vi "EF_GetFeaturesVectorScalogram.vi"(7 "TimeShiftsNum":dbl=50.0, 8 "ChannelNumber":i32=-1, 9 "High cutoff frequency":dbl, 10 "Low cutoff frequency":dbl, 11 "Array Of Waveforms in":waveform(dbl)[](array[waveform])) -> (0 "StackedSpectra":dbl[][](array[numeric]), 2 "size(s)":i32[](array[numeric]), 3 "StackedScalograms":dbl[][](array[numeric]))   [LabVIEW 2016, in "Feature Extraction.lvlib"]
uses:
  <vilib>/Analysis/baseanly.llb/Mean (DBL).vi
  <vilib>/addons/Wavelet Analysis/continuous wavelet transform.llb/WA Analytic Wavelet Transform (Waveform).vi
  Feature Extraction.lvlib
  <vilib>/addons/_Advanced Signal Processing/NI_AdvSigProcTFA.lvlib
  <vilib>/addons/_Advanced Signal Processing/NI_AdvSigProcWA.lvlib
  <vilib>/Analysis/NI_AALBase.lvlib
panel:
  out "Энергетический спектр сигнала ЭЭГ":dbl[](graph)
  out "Сигнал ЭЭГ":waveform(dbl)(graph)
  out "Матрица квадратов коэффициентов вейвлет-разложения":dbl[][](graph)
  # "This VI is a part of BCI Design library, http://www.ru-bci.org \nCopyright © 2020, Sotnikov Peter, All rights reserved. License: GNU GPLv3"
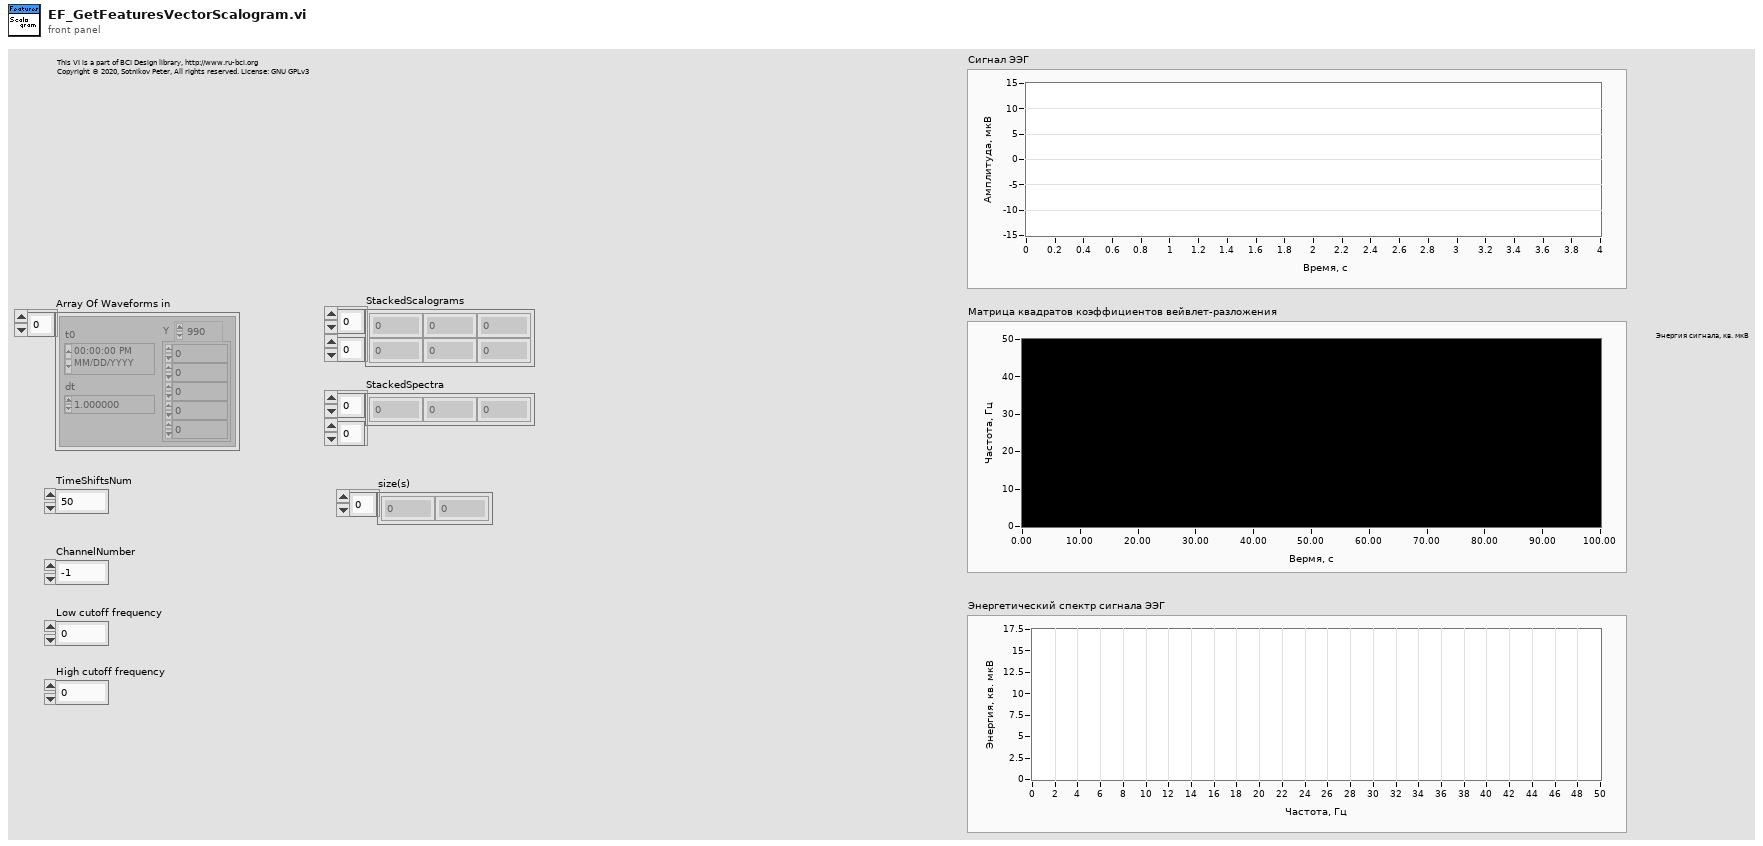
[diagram p1: front panel]
types:
  T1 = cluster{"frequency offset":dbl, "frequency multiplier":dbl}
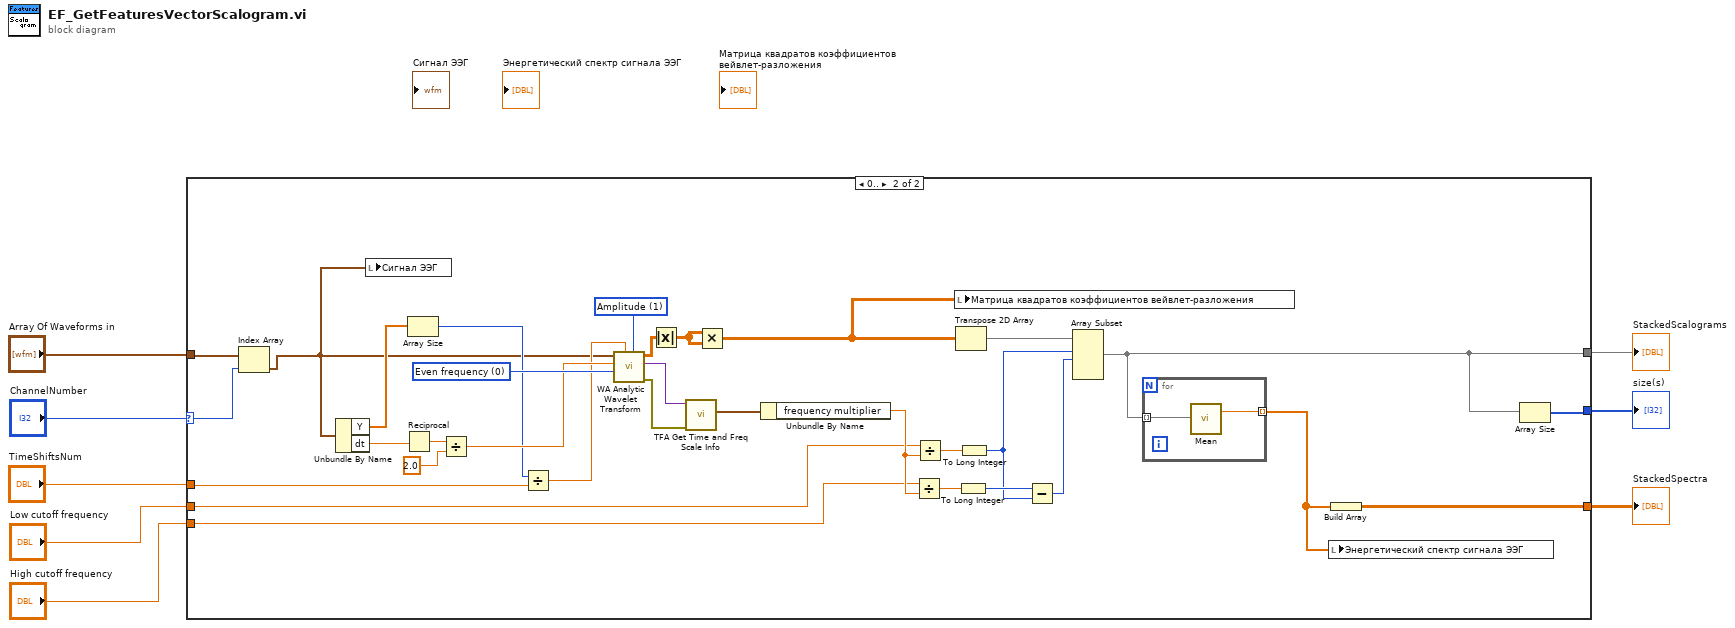
[diagram p0: block diagram]
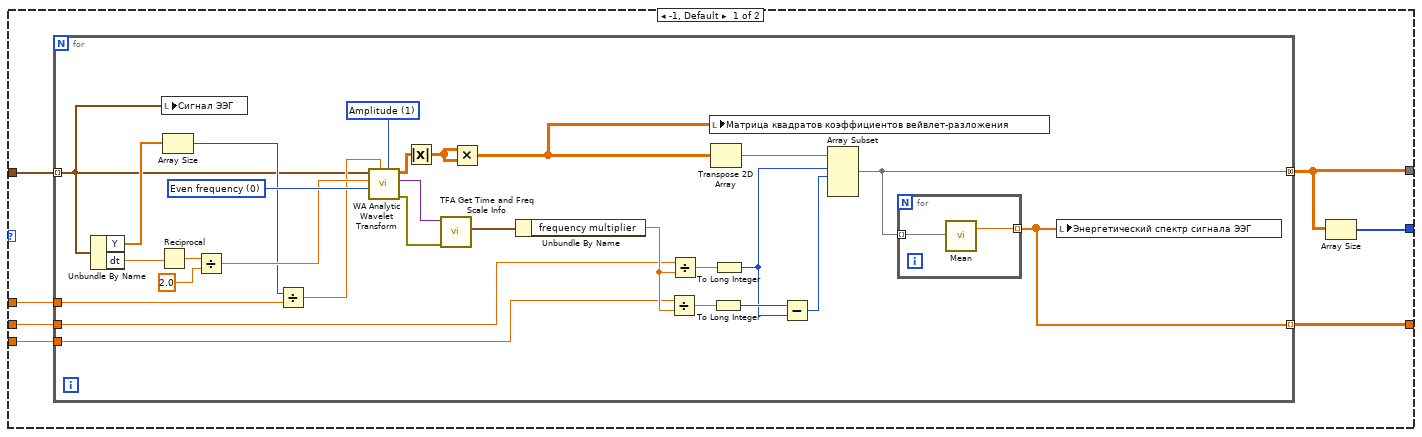
[diagram p2: hidden frame]
diagram:
  n1 = case shown="0.." "ChannelNumber" {
    selector: "ChannelNumber" -> [_ w56]
    tunnel: "Array Of Waveforms in" -> [w15 w57]
    tunnel: [w14 w50] -> w7
    tunnel: [w13 w51] -> w6
    tunnel: "TimeShiftsNum" -> [w12 w54]
    tunnel: [w11 w49] -> w4
    tunnel: "Low cutoff frequency" -> [w10 w47]
    tunnel: "High cutoff frequency" -> [w9 w46]
    frame -1, Default {
      n2 = for {
        tunnel: w15 -> [w20] mode=indexing
        tunnel: [w27] -> w14 mode=concatenating
        tunnel: w12 -> [w22]
        tunnel: [w18] -> w11 mode=indexing
        tunnel: w10 -> [w17]
        tunnel: w9 -> [w16]
        w40 = u16 0 items=["Even frequency", "Even scale"] ("scale sampling method")
        w41 = u16 1 items=["Energy", "Amplitude"] ("normalization")
        n3 = Unbundle By Name(w20) -> ("Y"=w30:dbl[], "dt"=w33:dbl)
        n4 = Reciprocal(x=w33) -> (1/x=w32:dbl)
        n5 = local write "Сигнал ЭЭГ"(w20) -> ()
        n6 = Array Size(array=w30) -> (size(s)=w21:i32)
        n7 = Divide(x=w32, y=2.0) -> (x/y=w24:dbl)
        n8 = Divide(x=w21, y=w22) -> (x/y=w23:dbl)
        n9 = call-poly <vilib>:"WA Analytic Wavelet Transform.vi"("normalization"=w41, "time steps"=w23, "scale sampling method"=w40, "scales"=w24, "signal"=w20) -> ("error out"=w43:errorcluster, "scale info"=w28:variant, "AWT coef"=w26:cdb[][])  [unwired: 4 in]
        n10 = Absolute Value(x=w26) -> (abs(x)=w25:dbl[][])
        n11 = call <vilib>:"TFA Get Time and Freq Scale Info.vi"("error in (no error)"=w43, "scale info"=w28) -> ("frequency info"=w42:T1)  [unwired: 7 in, 2 out]
        n12 = Multiply(x=w25, y=w25) -> (x*y=w19:dbl[][])
        n13 = Unbundle By Name(w42) -> ("frequency multiplier"=w37:dbl)
        n14 = Divide(x=w16, y=w37) -> (x/y=w39:dbl)
        n15 = Divide(x=w17, y=w37) -> (x/y=w38:dbl)
        n16 = local write "Матрица квадратов коэффициентов вейвлет-разложения"(w19) -> ()
        n17 = Transpose 2D Array(2D array=w19) -> (transposed array=w29:dbl[][])
        n18 = To Long Integer(number=w39) -> (32bit integer=w36:i32)
        n19 = To Long Integer(number=w38) -> (32bit integer=w35:i32)
        n20 = Subtract(x=w36, y=w35) -> (x-y=w34:i32)
        n21 = Array Subset(array=w29, index (row)=w35, length (row)=w34) -> (w27:dbl[][])  [unwired: 2 in]
        n22 = for {
          tunnel: w27 -> [w45] mode=indexing
          tunnel: [w44] -> w18 mode=indexing
          n23 = call-poly <vilib>:"Mean.vi"("X"=w45) -> ("mean"=w44:dbl)  [unwired: 1 out]
        }
        n24 = local write "Энергетический спектр сигнала ЭЭГ"(w18) -> ()
      }
      n25 = Array Size(array=w14) -> (size(s)=w13:i32[])
    }
    frame 0.. {
      w53 = u16 1 items=["Energy", "Amplitude"] ("normalization")
      w75 = u16 0 items=["Even frequency", "Even scale"] ("scale sampling method")
      n26 = Index Array(array=w57, index=w56) -> (element=w55:waveform(dbl))
      n27 = Unbundle By Name(w55) -> ("Y"=w65:dbl[], "dt"=w68:dbl)
      n28 = local write "Сигнал ЭЭГ"(w55) -> ()
      n29 = Reciprocal(x=w68) -> (1/x=w67:dbl)
      n30 = Array Size(array=w65) -> (size(s)=w58:i32)
      n31 = Divide(x=w67, y=2.0) -> (x/y=w60:dbl)
      n32 = Divide(x=w58, y=w54) -> (x/y=w59:dbl)
      n33 = call-poly <vilib>:"WA Analytic Wavelet Transform.vi"("normalization"=w53, "time steps"=w59, "scale sampling method"=w75, "scales"=w60, "signal"=w55) -> ("error out"=w77:errorcluster, "scale info"=w63:variant, "AWT coef"=w62:cdb[][])  [unwired: 4 in]
      n34 = Absolute Value(x=w62) -> (abs(x)=w61:dbl[][])
      n35 = call <vilib>:"TFA Get Time and Freq Scale Info.vi"("error in (no error)"=w77, "scale info"=w63) -> ("frequency info"=w76:T1)  [unwired: 7 in, 2 out]
      n36 = Multiply(x=w61, y=w61) -> (x*y=w52:dbl[][])
      n37 = Unbundle By Name(w76) -> ("frequency multiplier"=w72:dbl)
      n38 = Divide(x=w46, y=w72) -> (x/y=w74:dbl)
      n39 = Divide(x=w47, y=w72) -> (x/y=w73:dbl)
      n40 = local write "Матрица квадратов коэффициентов вейвлет-разложения"(w52) -> ()
      n41 = Transpose 2D Array(2D array=w52) -> (transposed array=w64:dbl[][])
      n42 = To Long Integer(number=w74) -> (32bit integer=w71:i32)
      n43 = To Long Integer(number=w73) -> (32bit integer=w70:i32)
      n44 = Subtract(x=w71, y=w70) -> (x-y=w69:i32)
      n45 = Array Subset(array=w64, index (row)=w70, length (row)=w69) -> (w50:dbl[][])  [unwired: 2 in]
      n46 = for {
        tunnel: w50 -> [w79] mode=indexing
        tunnel: [w78] -> w48 mode=indexing
        n47 = call-poly <vilib>:"Mean.vi"("X"=w79) -> ("mean"=w78:dbl)  [unwired: 1 out]
      }
      n48 = local write "Энергетический спектр сигнала ЭЭГ"(w48) -> ()
      n49 = Build Array(w48) -> (w49:dbl[][])
      n50 = Array Size(array=w50) -> (size(s)=w51:i32[])
    }
  }
  "StackedScalograms" <- w7
  "size(s)" <- w6
  "StackedSpectra" <- w4
